vi "X-absolute_position.vi"(11 ".NET Refnum in":refnum<k24>) -> (2 "Numeric":dbl format="%#.6g", 3 ".NET Refnum out":refnum<k24>)   [LabVIEW 2021]
uses:
  C:/Users/User/Documents/Published_files/thorlabs_files/Thorlabs.MotionControl.IntegratedStepperMotorsCLI.dll
  thorlabs_files/Thorlabs.MotionControl.IntegratedStepperMotorsCLI.dll
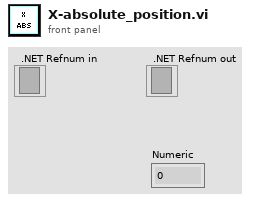
[diagram p1: front panel]
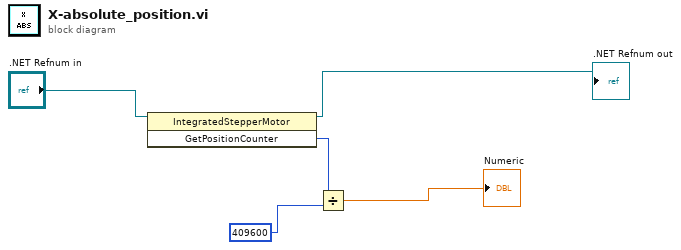
[diagram p0: block diagram]
diagram:
  n1 = invoke class="IntegratedStepperMotor" method="GetPositionCounter"(reference=".NET Refnum in") -> (reference out=→".NET Refnum out":refnum<k24>, "GetPositionCounter"=w3:i32)  [unwired: 2 in, 1 out]
  n2 = Divide(x=w3, y=409600) -> (x/y=→"Numeric":dbl)
